vi "Write States.vi"(8 "error in (no error)":errorcluster, 10 "States":T1=enum."Exit", 11 "KickToBestRobotTactic in":refnum<class "KickToBestRobotTactic.lvclass">) -> (0 "error out":errorcluster, 3 "KickToBestRobotTactic out":refnum<class "KickToBestRobotTactic.lvclass">)   [LabVIEW 2024, in "KickToBestRobotTactic.lvclass"]
uses:
  KickToBestRobotTactic.lvclass
  KickTOBestRobotTacticStatesEnum.ctl
  KickToBestRobotTactic.lvclass/KickToBestRobotTactic.ctl
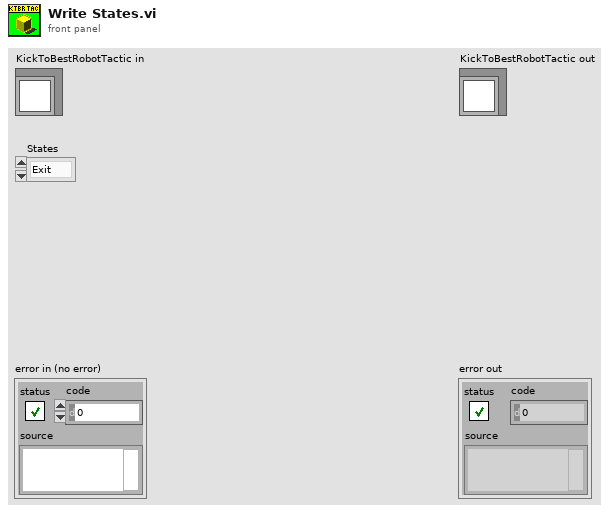
[diagram p1: front panel]
types:
  T1 = typedef "KickToBestRobotTactic.lvclass/KickTOBestRobotTacticStatesEnum.ctl" = enum16{"WaitToPass", "Pass", "Exit"}
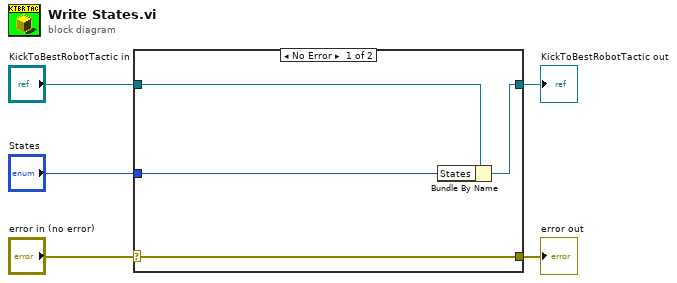
[diagram p0: block diagram]
diagram:
  n1 = case shown="No Error" "error in (no error)" {
    selector: "error in (no error)" -> [w9 w10]
    tunnel: [w9 w10] -> w4
    tunnel: [w7 w11] -> w2
    tunnel: "KickToBestRobotTactic in" -> [w8 w11]
    tunnel: "States" -> [w6 _]
    frame No Error {
      n2 = Bundle By Name(cluster=w8, "States"=w6) -> (w7:refnum<class "KickToBestRobotTactic.lvclass">)
    }
    frame Error {
    }
  }
  "error out" <- w4
  "KickToBestRobotTactic out" <- w2
